vi "LEP_RV_ConcatenateLastWords.vi"(10 "Initial array length":i32, 11 "Inittial array":string[](array[string])) -> (3 "Array containing exactly 7 words":string[](array[string]))   [LabVIEW 2011]
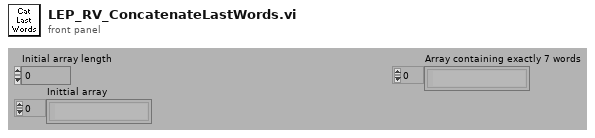
[diagram p1: front panel]
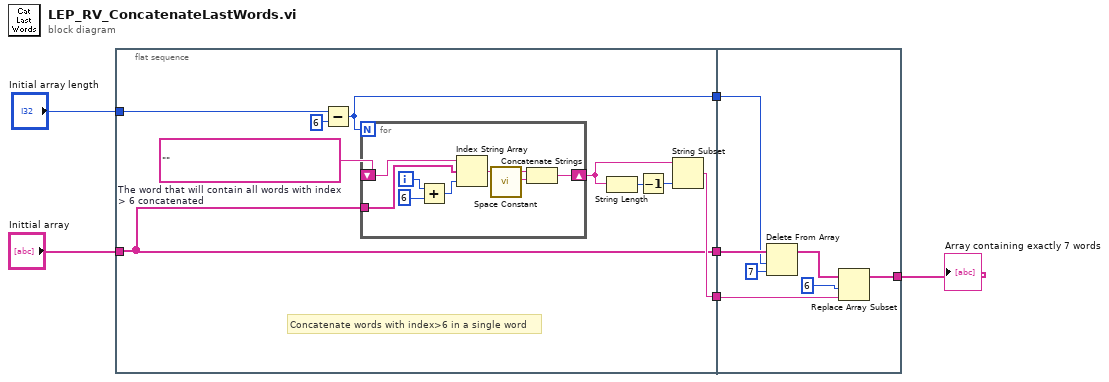
[diagram p0: block diagram]
diagram:
  n1 = flat-sequence {
    tunnel: "Initial array length" -> [w15]
    tunnel: "Inittial array" -> [w7]
    tunnel: [w7] -> w6
    tunnel: [w12] -> w2
    tunnel: [w8] -> w1
    tunnel: w6 -> [w28]
    tunnel: [w30] -> w3
    tunnel: w2 -> [w29]
    tunnel: w1 -> [w26]
    frame #0 {
      w13 = ""  # The word that will contain all words with index > 6 concatenated
      # "Concatenate words with index>6 in a single word"
      n2 = Subtract(x=w15, y=6) -> (x-y=w8:i32)
      n3 = for {
        N: w8 -> [_]
        shift-right: [w16] -> w11
        shift-left: w13 -> [w23]
        tunnel: w7 -> [w19]
        i -> [w22]
        n4 = Add(x=w22, y=6) -> (x+y=w20:i32)
        n5 = Index String Array(1:w20, 2:w19, 3:w23) -> (0:w18:string)
        n6 = call <vilib>:"Space Constant.vi"() -> ("String"=w17:string)
        n7 = Concatenate Strings(w18, w17) -> (w16:string)
      }
      n8 = String Length(string=w11) -> (length=w10:i32)
      n9 = Decrement(x=w10) -> (x-1=w9:i32)
      n10 = String Subset(string=w11, length (rest)=w9) -> (substring=w12:string)  [unwired: 1 in]
    }
    frame #1 {
      n11 = Delete From Array(array=w28, length=w26, index=7) -> (array with subset deleted=w24:string[])  [unwired: 1 out]
      n12 = Replace Array Subset(array=w24, new element=w29, index=6) -> (w30:string[])
    }
  }
  "Array containing exactly 7 words" <- w3
